vi "Shutdown.vi"(8 "error in (no error)":errorcluster, 11 "Plugin in":refnum<class "Plugin.lvclass">) -> (0 "error out":errorcluster, 3 "Plugin out":refnum<class "Plugin.lvclass">)   [LabVIEW 2017, in "Data Sharing Framework Core.lvlib" / "Data Sharing Framework Engine.lvlib" / "Plugin.lvclass"]
uses:
  Plugin.lvclass
  Plugin.lvclass/Plugin.ctl
  Internal/Transceiver/Transceiver Thread/Transceiver Thread.lvclass
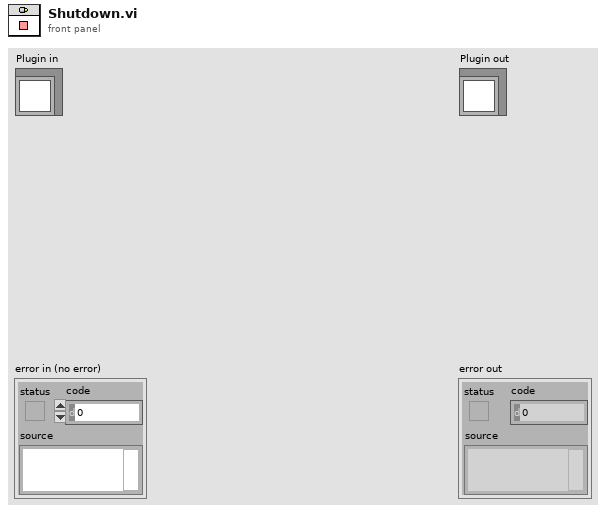
[diagram p1: front panel]
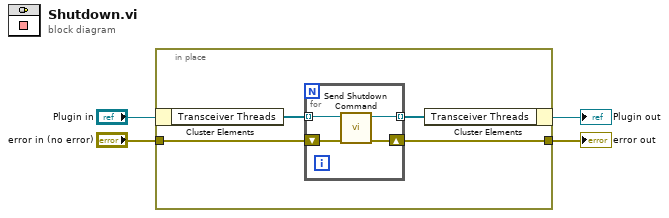
[diagram p0: block diagram]
diagram:
  n1 = in-place {
    in-place-border: "error in (no error)" -> [w8]
    in-place-border: [w7] -> w1
    n2 = in-place-cluster #1("Plugin in") -> ("Transceiver Threads"=w6:refnum<class "Transceiver Interface.lvclass">[])
    n3 = for {
      shift-right: [w9] -> w7
      shift-left: w8 -> [w10]
      tunnel: [w11] -> w5 mode=indexing
      tunnel: w6 -> [w12] mode=indexing
      n4 = call "Send Shutdown Command.vi"("error in (no error)"=w10, "Transceiver Interface in"=w12) -> ("error out"=w9:errorcluster, "Transceiver Interface out"=w11:refnum<class "Transceiver Interface.lvclass">)  [unwired: 8 in]
    }
    n5 = in-place-cluster #1("Transceiver Threads"=w5) -> (→"Plugin out":refnum<class "Plugin.lvclass">)
  }
  "error out" <- w1
